vi "Multi-Loop Humidity Control.vi"(4 "Reset?":bool, 5 "dTmax":dbl=1.0 format="%#_13g", 6 "dt (s)":dbl=2.0, 7 "PID":T1(array[cluster]) {"derivative time (Td, min)" format="%.3f"; "integral time (Ti, min)" format="%.3f"; "proportional gain (Kc)" format="%.3f"}, 8 "error in":errorcluster, 9 "TspIn":dbl[](array[numeric]) format="%#.2g", 10 "RH meas":dbl[](array[numeric]) format="%.2f", 11 "RHsp":dbl[](array[numeric]) format="%.2f") -> (0 "error out":errorcluster, 2 "PID Out":sgl[](array[numeric]) format="%.2f", 3 "TspOut":sgl[](array[numeric]) format="%.2f")   [LabVIEW 2015]
doc: "This VI updates the temperature setpoint on the UHSAS RH control system using a PID algorithm. For this algortihm:\n* The error, e, is RHsp - RHmeas\n* The output of the control loop is u. This variable is transformed to temperature by associating it with an assumed saturator efficieny. Ideally, the saturator efficiency is 1, but there may be uncertainties that limit this. There fore, the output u, is transformed to an efficiency k by using the following assumptions:\n * when RHmeas < RHsp, k <1\n * when RHmeas > RHsp, k >1\n * when RHmeas = RHsp, k = 1\n To relate temperature to this k, we assume that the k*RHcal= k*esat(Tsp)/esat(Tair)=RHmeas. From this equation, we can calculate the dewpoint of the air exiting the saturator based on the efficiency term k \n* The dewpoint calculated above is the new saturator setpoint."
uses:
  <vilib>/addons/control/pid/pid.llb/PID (DBL Array).vi
  <vilib>/addons/control/pid/NI_PID_pid.lvlib
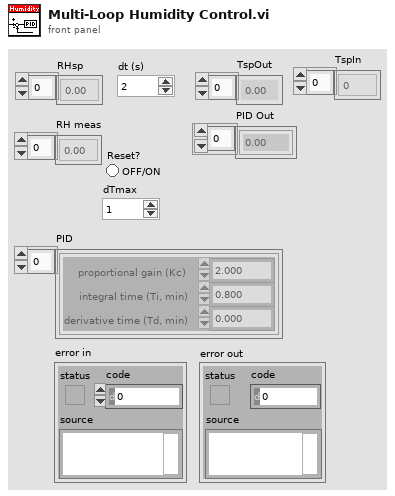
[diagram p1: front panel]
types:
  T1 = cluster{"proportional gain (Kc)":dbl, "integral time (Ti, min)":dbl, "derivative time (Td, min)":dbl}[]
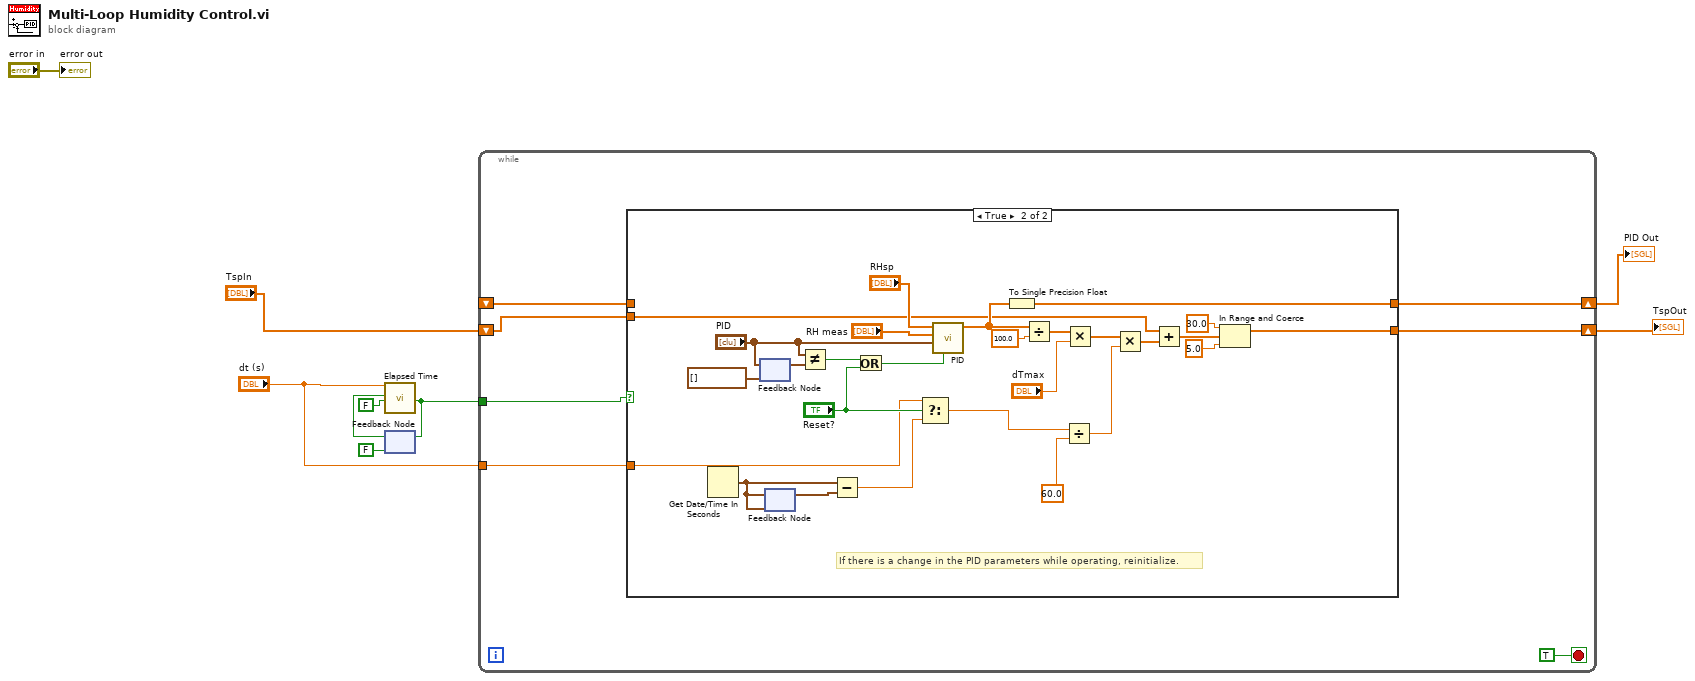
[diagram p0: block diagram]
diagram:
  n1 = feedback #1(FALSE ("Time has Elapsed")) -> (w7:bool)
  n2 = call "Elapsed Time"("Time Target (s)"="dt (s)", "Reset"=w7, "Auto Reset"=FALSE) -> ("Time has Elapsed"=w3:bool)  [unwired: 9 in, 7 out]
  n3 = feedback-in #1(w3) -> ()
  n4 = while {
    shift-right: [w16] -> w5
    shift-left: "TspIn" -> [w15]
    tunnel: w3 -> [w14]
    shift-right: [w12] -> w2
    shift-left: _ -> [w11]
    tunnel: "dt (s)" -> [w10]
    stop <- TRUE stop-if-true
    n5 = case shown="True" w14 {
      tunnel: [w18 w25] -> w16
      tunnel: w15 -> [w18 w24]
      tunnel: [w17 w23] -> w12
      tunnel: w11 -> [w17 _]
      tunnel: w10 -> [_ w20]
      frame False {
      }
      frame True {
        # "If there is a change in the PID parameters while operating, reinitialize."
        n6 = Get Date/Time In Seconds() -> (seconds since 1Jan1904=w34:timestamp)
        n7 = feedback #2(T1 []) -> (w45:T1)
        n8 = feedback-in #2("PID") -> ()
        n9 = feedback #3(w34) -> (w33:timestamp)
        n10 = feedback-in #3(w34) -> ()
        n11 = Not Equal?(x="PID", y=w45) -> (x != y?=w40:bool)
        n12 = Subtract(x=w34, y=w33) -> (x-y=w21:dbl)
        n13 = Or(x=w40, y="Reset?") -> (x .or. y?=w39:bool)
        n14 = Select(t=w20, s="Reset?", f=w21) -> (s? t:f=w19:dbl)
        n15 = call-poly <vilib>:"PID.vi"("reinitialize? (F)"=w39, "PID gains"="PID", "process variable"="RH meas", "setpoint"="RHsp") -> ("output"=w38:dbl[])  [unwired: 6 in, 1 out]
        n16 = To Single Precision Float(number=w38) -> (single precision float=w23:sgl[])
        n17 = Divide(x=w38, y=100.0) -> (x/y=w36:dbl[])
        n18 = Divide(x=w19, y=60.0) -> (x/y=w31:dbl)
        n19 = Multiply(x=w36, y="dTmax") -> (x*y=w30:dbl[])
        n20 = Multiply(x=w30, y=w31) -> (x*y=w29:dbl[])
        n21 = Add(x=w24, y=w29) -> (x+y=w28:dbl[])
        n22 = In Range and Coerce(upper limit=30.0, x=w28, lower limit=5.0) -> (coerced(x)=w25:dbl[])  [unwired: 1 out]
      }
    }
  }
  "TspOut" <- w5
  "PID Out" <- w2
  "error out" <- "error in"
